vi "GV DO0.vi"() -> ()   [LabVIEW 2017]
panel:
  out "DO0":bool
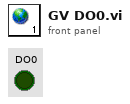
[diagram p1: front panel]
diagram:
